vi "Get Channel Name.vi"(0 "Pin Name[]":string[](array[string]), 5 "session reservation in":refnum<class "Session Reservation.lvclass">, 11 "error in (no error)":errorcluster) -> (4 "Channel Name":string[](array[string]), 6 "Channel Number":string[](array[string]), 8 "Session Exists":bool[](array[boolean]), 10 "Session.name":string[](array[string]), 15 "error out":errorcluster)   [LabVIEW 2024, in "devicePowerSequencerCoreLogic.lvlib"]
uses:
  devicePowerSequencerCoreLogic.lvlib
  <vilib>/Plug-In SDKs/Clients/Session Management V1/Session Reservation/Session Reservation.lvclass
  <vilib>/Plug-In SDKs/Sessions/niDCPower/Get Connections - 1Pin 1Conn.vi
  <vilib>/Plug-In SDKs/Sessions/niDCPower/NI Session Management niDCPower.lvlib
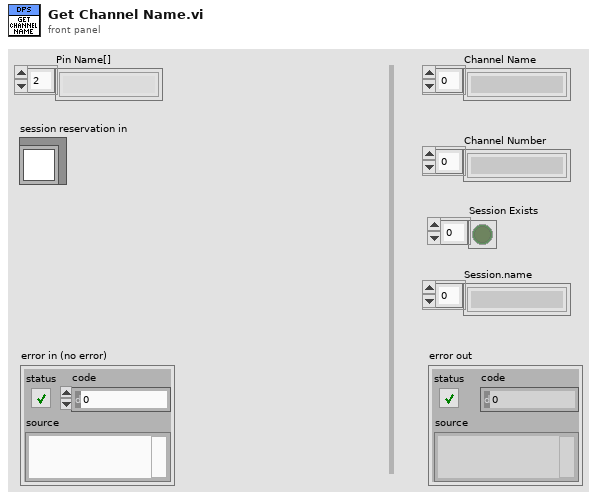
[diagram p1: front panel]
types:
  T1 = typedef "NI Session Management niDCPower.lvlib/Connection with Session.ctl" = cluster{"connection":T2, "session":refnum<k15>}
  T2 = typedef "NI Session Management V1 Client.lvlib/Session Reservation.lvclass/Connection.ctl" = cluster{"pin or relay name":string, "site":i32, "instrument type id":string, "channel":string}
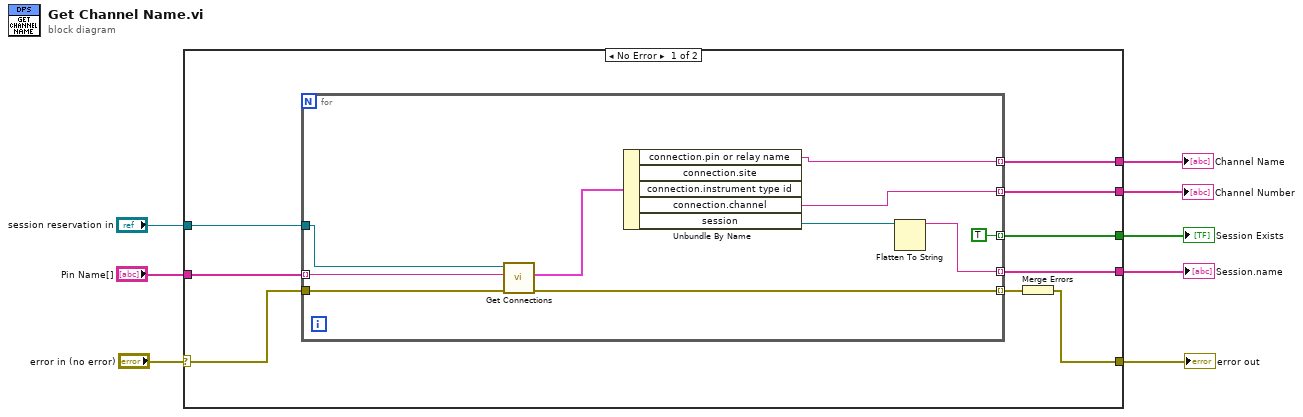
[diagram p0: block diagram]
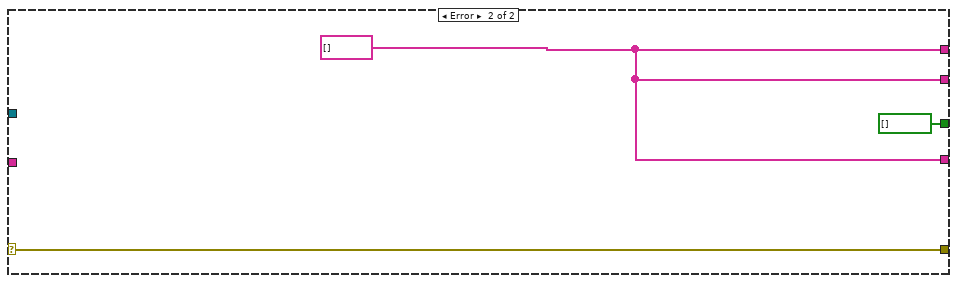
[diagram p2: hidden frame]
diagram:
  n1 = case shown="No Error" "error in (no error)" {
    selector: "error in (no error)" -> [w12 w30]
    tunnel: "Pin Name[]" -> [w17 _]
    tunnel: [w10 w30] -> w6
    tunnel: [w16 w28] -> w5
    tunnel: [w15 w28] -> w4
    tunnel: [w14 w28] -> w3
    tunnel: [w13 bool[] []] -> w2
    tunnel: "session reservation in" -> [w9 _]
    frame No Error {
      n2 = for {
        tunnel: w17 -> [w27] mode=indexing
        tunnel: [w25] -> w16 mode=indexing
        tunnel: [w24] -> w15 mode=indexing
        tunnel: [w22] -> w14 mode=indexing
        tunnel: [TRUE] -> w13 mode=indexing
        tunnel: w12 -> [w20]
        tunnel: [w19] -> w11 mode=indexing
        tunnel: w9 -> [w18]
        n3 = call-poly <vilib>:"Get Connections.vi"("error in"=w20, "pin or relay name"=w27, "session reservation in"=w18) -> ("error out"=w19:errorcluster, "connection"=w26:T1)  [unwired: 6 in, 1 out]
        n4 = Unbundle By Name(w26) -> ("connection.pin or relay name"=w25:string, "connection.channel"=w24:string, "session"=w23:refnum<k15>)  [unwired: 2 out]
        n5 = Flatten To String(anything=w23) -> (data string=w22:string)  [unwired: 3 in, 2 out]
      }
      n6 = Merge Errors(w11) -> (w10:errorcluster)
    }
    frame Error {
      w28 = string[] []
    }
  }
  "error out" <- w6
  "Channel Name" <- w5
  "Channel Number" <- w4
  "Session Exists" <- w2
  "Session.name" <- w3
